vi "check for timeout.vi"(8 "error in (no error)":errorcluster, 11 "Data Value Reference in":refnum<data-value>) -> (0 "error out":errorcluster)   [LabVIEW 2015, in "Modbus Master Engine.lvlib"]
uses:
  Modbus Master Engine.lvlib
  <vilib>/addons/Inline Async API/_Data Access Engine/Access Type Classes/Write/Write.lvclass
  <vilib>/addons/Inline Async API/_Data Access Engine/Access Type Classes/Write/Write.lvclass/Write.ctl
  <vilib>/addons/Inline Async API/_Data Access Engine/Data Access Engine/Methods/Write.Data.vi
  <vilib>/addons/Inline Async API/_Data Access Engine/Access Type Classes/Write/Write.ProcessData.vi
  <vilib>/addons/Inline Async API/_Data Access Engine/Data Access Engine/Data Access Engine.lvclass
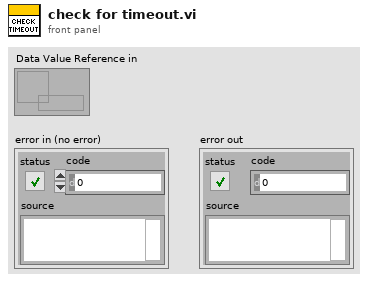
[diagram p1: front panel]
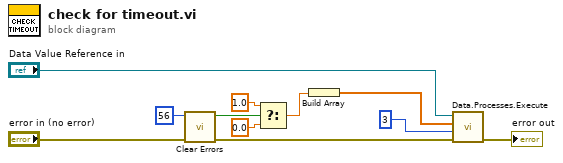
[diagram p0: block diagram]
diagram:
  n1 = call <vilib>:"Clear Errors.vi"("error in (no error)"="error in (no error)", "specific error code to clear (0: all)"=56) -> ("error out"=w3:errorcluster, "specific error cleared?"=w1:bool)  [unwired: 4 in]
  n2 = Select(t=1.0 ("Channel Data Reference"), s=w1, f=0.0) -> (s? t:f=w5:dbl)
  n3 = Build Array(w5) -> (w8:dbl[])
  n4 = call-poly <vilib>:"Data.Processes.Execute.vi"("error in (no error)"=w3, "Offset"=3, "Values"=w8, "Ref"="Data Value Reference in") -> ("error out"=→"error out":errorcluster)  [unwired: 7 in]
